vi "通道配置模块.vi"() -> (1 "返回":bool)   [LabVIEW 2010]
uses:
  全局量/试验配置信息.vi
  全局量/全局_配置.vi
  <vilib>/Utility/config.llb/Write Key (String).vi
  <vilib>/Utility/config.llb/NI_LVConfig.lvlib
panel:
  in  "str_IP":string
  in  "单选_LAN":bool
  in  "CAN波特率":T1(ring)
  in  "LAN端口":u32
  in  "RS485_2端口":refnum<visa-resource-name>="COM1"
  in  "RS485_1端口":refnum<visa-resource-name>="COM1"
  in  "RS485波特率":T2(ring)
  in  "R232端口":refnum<visa-resource-name>="COM1"
  out "配置文件路径":path
  out "配置文件目录":path
  in  "btn_保存配置":bool
  in  "加载配置文件列表":u16(ring)
  in  "保存配置文件名称":string
  in  "btn_返回":bool
  in  "选项卡控件":T3(tab)
  in  "CAN路数":u32=1 min=1 max=4
  in  "RS485路数":u32=1 min=1 max=1
  in  "RS232路数":u32=1 min=1 max=2
  in  "AD输入幅值":enum32{"±3V", "±5V", "±12V"}(ring)
  in  "AD输入路数":u32 min=1 max=16
  in  "DSP输入幅值":enum32{"0-3V"}(ring)
  in  "DSP输入路数":u32 min=1 max=16
  in  "数字量输入路数":u32 min=1 max=80
  in  "模拟量误差":dbl format="%.4f"
  in  "数字量输出路数":u32=1 min=1 max=76
  in  "D_IN_1":string[][](table) caption="表格"
  in  "D_IN_2":string[][](table) caption="表格"
  in  "D_IN_3":string[][](table) caption="表格"
  in  "D_IN_4":string[][](table) caption="表格"
  # "板卡测试配置"
  # "保存配置文件名称："
  # "加载配置文件："
  # "控制板IP："
  # "控制板端口："
  # "1号"
  # "COM端口："
  # "2号"
  # "COM端口："
  # "CAN总线通信波特率："
  # "RS485总线通信波特率："
  # "数字量输出信号路数："
  # "数字量输入信号路数："
  # "外部AD模拟量输入信号路数："
  # "DSP模拟量输入信号路数："
  # "外部AD模拟量输入信号幅值："
  # "DSP模拟量输入信号幅值："
  # "RS232总线通信路数："
  # "RS485总线通信路数："
  # "CAN总线通信路数："
  # "模拟量允许误差："
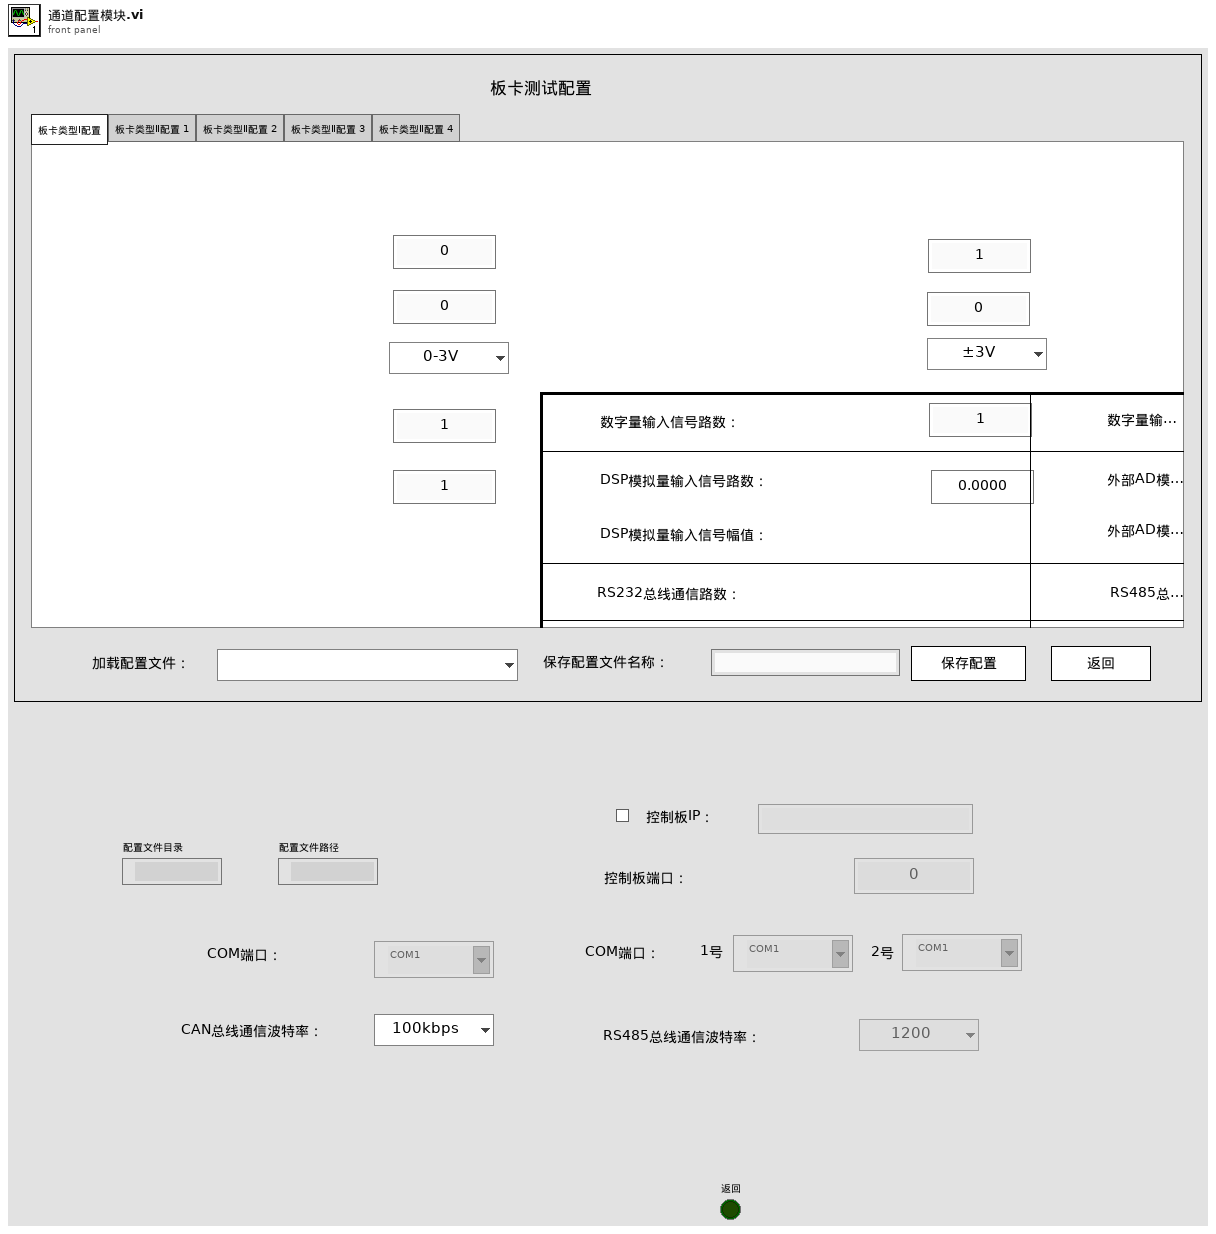
[diagram p1: front panel]
types:
  T1 = enum32{"100kbps", "200kbps", "250kbps", "500kbps", "1000kbps"}
  T2 = enum32{"1200", "2400", "4800", "9600", "19200", "57600", "115200", ""}
  T3 = enum32{"板卡类型Ⅰ配置", "板卡类型Ⅱ配置 1", "板卡类型Ⅱ配置 2", "板卡类型Ⅱ配置 3", "板卡类型Ⅱ配置 4"}
  T4 = enum8{"Enabled", "Disabled", "Disabled and Grayed Out"}
  T5 = cluster{"数字量输入路数":u32, "数字量输出路数":u32, "DSP输入路数":u32, "DSP输入幅值":enum32{"0-3V"}, "AD输入路数":u32, "AD输入幅值":enum32{"±3V", "±5V", "±12V"}, "毫秒倍数":u32, "RS232路数":u32, "模拟量误差":dbl, "毫秒倍数":u32, "RS485路数":u32, "RS485波特率":enum32{"1200", "2400", "4800", "9600", "19200", "57600", "115200", ""}, "CAN路数":u32, "CAN波特率":enum32{"100kbps", "200kbps", "250kbps", "500kbps", "1000kbps"}, "单选_LAN":bool, "str_IP":string, "LAN端口":u32}
  T6 = typedef "NI_LVConfig.lvlib/Config Data RefNum.ctl" = refnum<k1>
  T7 = cluster{"数字量输入信号路数":i32, "数字量输出信号路数":i32, "DSP模拟量输入信号路数":u32, "DSP模拟量输入信号幅值":u32, "AD模拟量输入信号路数":u32, "AD模拟量输入信号幅值":u32, "RS232端口":u32, "RS232通信路数":u32, "RS232波特率":dbl, "RS485端口":u32, "RS485通信路数":u32, "RS485波特率":u32, "CAN通信路数":i32, "CAN波特率":u32, "以太网选择?":bool, "控制板IP":string, "以太网端口":u32}
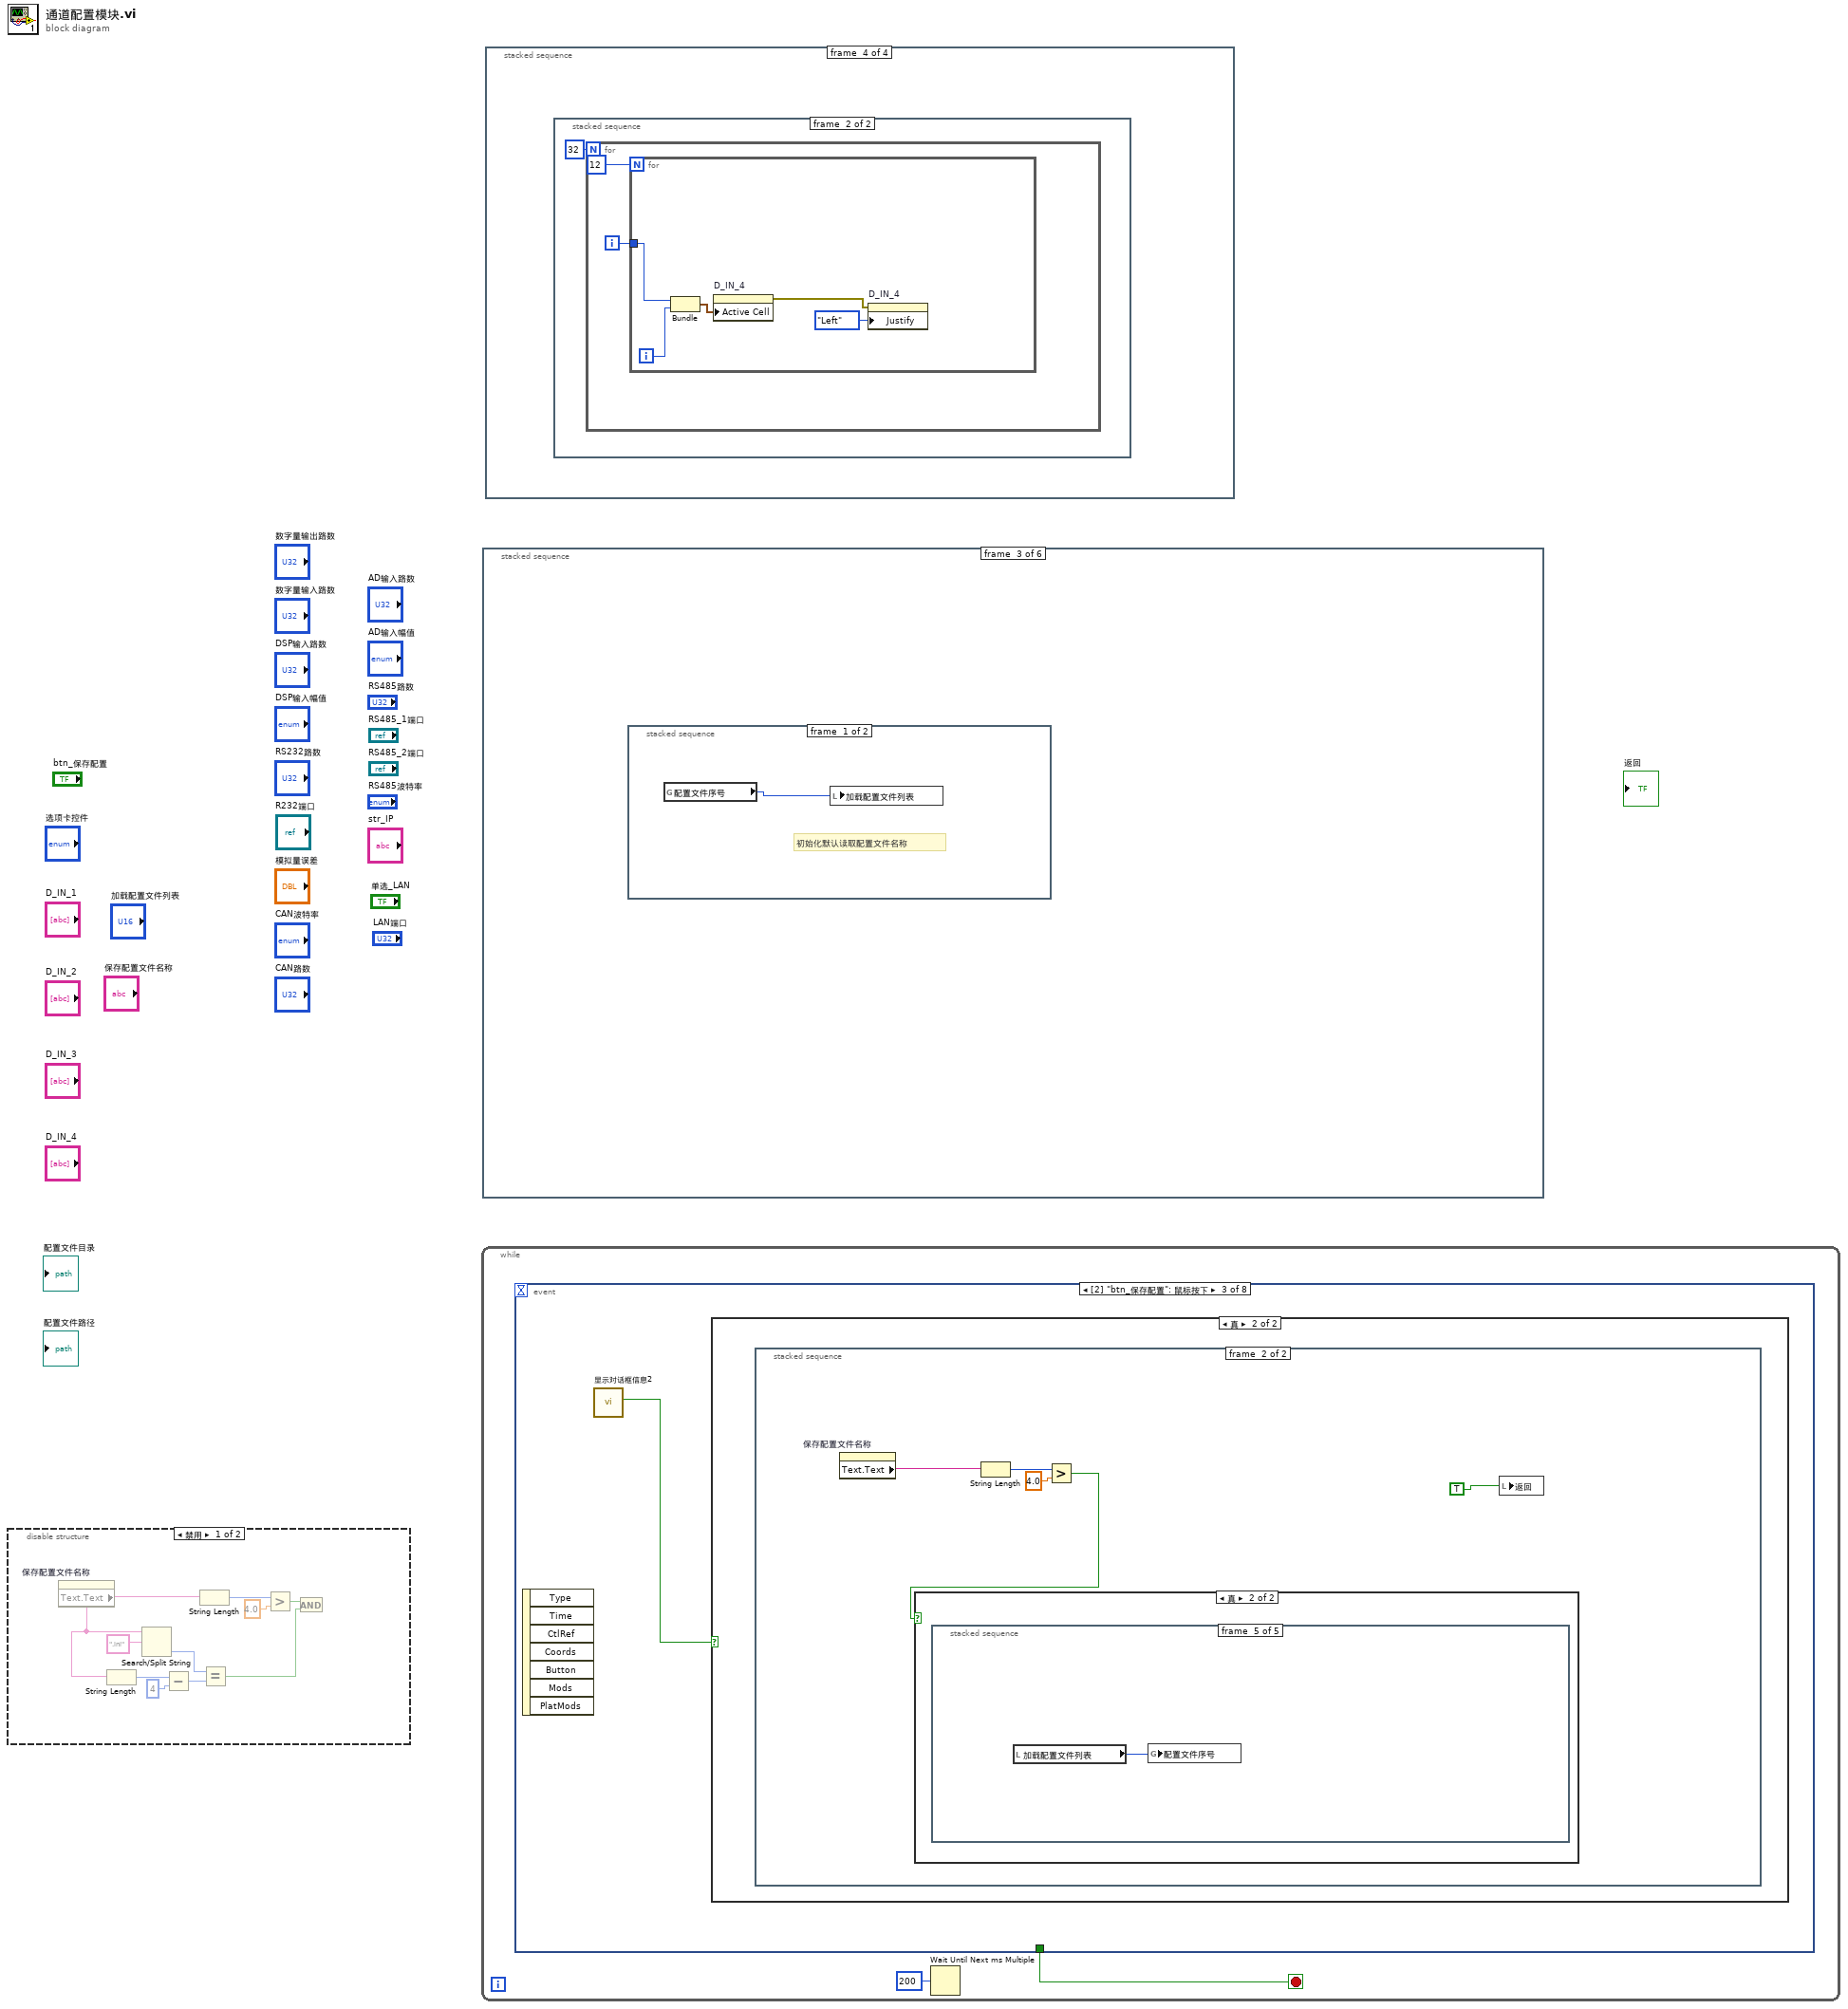
[diagram p0: block diagram]
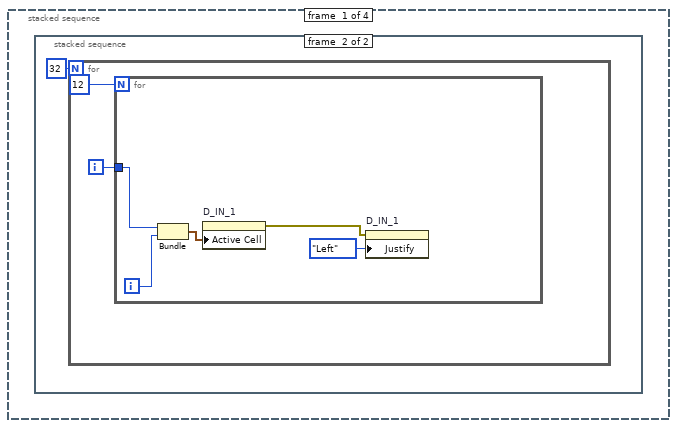
[diagram p2: hidden frame]
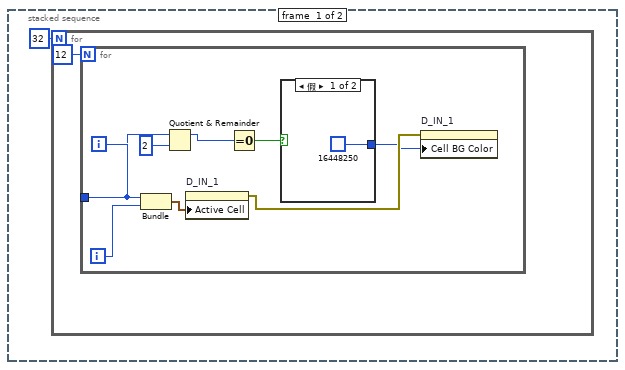
[diagram p3: hidden frame]
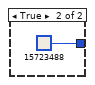
[diagram p4: hidden frame]
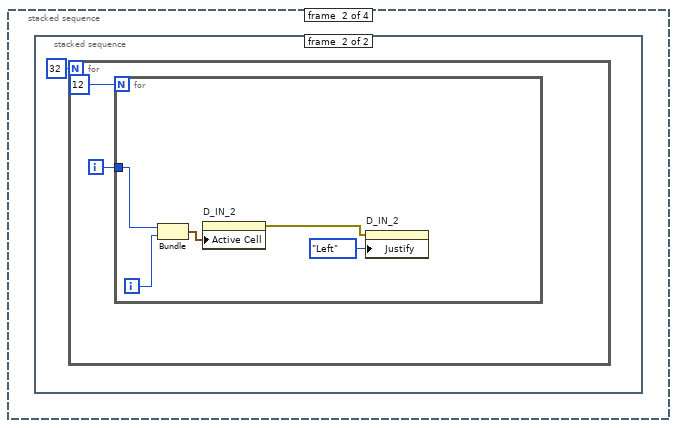
[diagram p5: hidden frame]
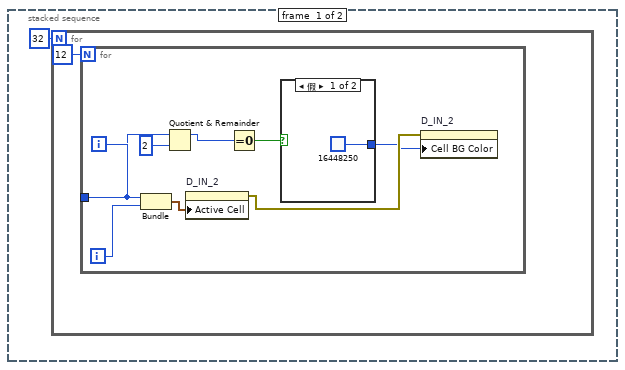
[diagram p6: hidden frame]
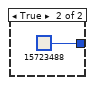
[diagram p7: hidden frame]
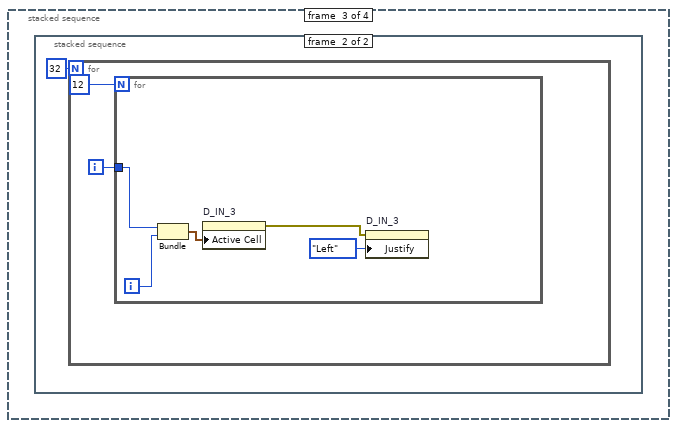
[diagram p8: hidden frame]
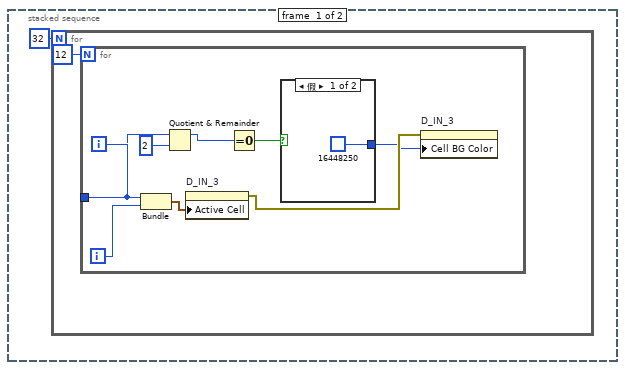
[diagram p9: hidden frame]
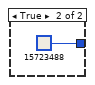
[diagram p10: hidden frame]
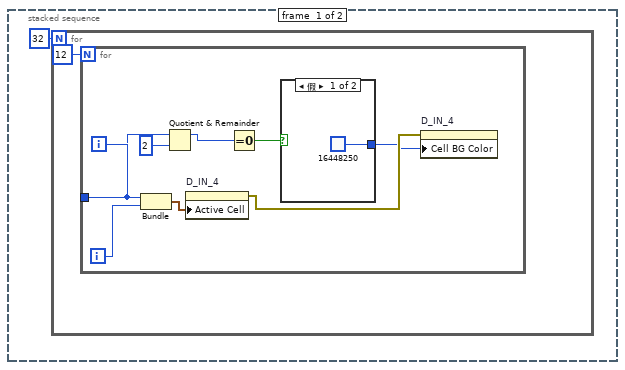
[diagram p11: hidden frame]
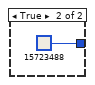
[diagram p12: hidden frame]
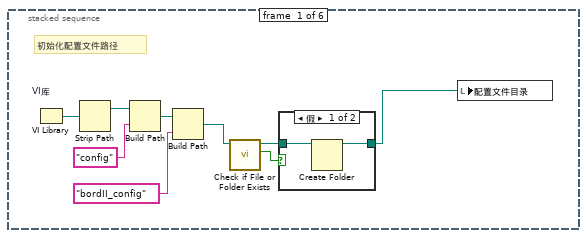
[diagram p14: hidden frame]
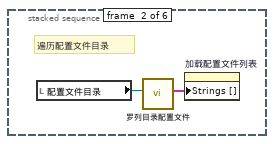
[diagram p16: hidden frame]
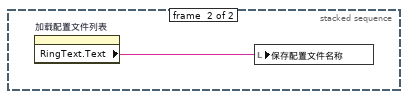
[diagram p17: hidden frame]
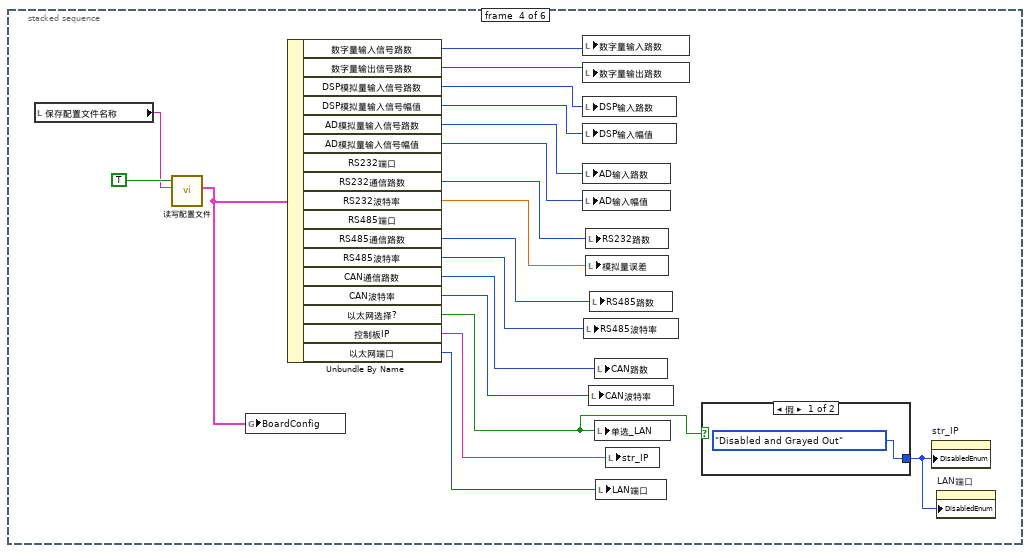
[diagram p18: hidden frame]
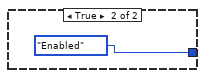
[diagram p19: hidden frame]
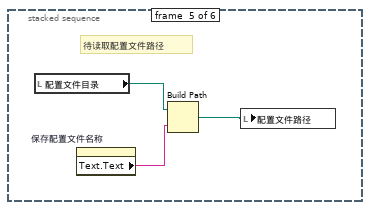
[diagram p20: hidden frame]
diagram:
  n1 = disable-structure shown="禁用" {
    frame Disabled {
      n2 = property on="保存配置文件名称" class="Str"() -> ("Text.Text"=w6:string)  [unwired: 2 in, 2 out]
      n3 = String Length(string=w6) -> (length=w7:i32)
      n4 = Search/Split String(string=w6, search string/char (-)=".ini" ("搜索字符串/字符(-)")) -> (offset of match=w5:i32)  [unwired: 1 in, 2 out]
      n5 = Subtract(x=w7, y=4) -> (x-y=w9:i32)
      n6 = String Length(string=w6) -> (length=w3:i32)
      n7 = Equal?(x=w5, y=w9) -> (x = y?=w10:bool)
      n8 = Greater?(x=w3, y=4.0) -> (0:w4:bool)
      n9 = And(x=w4, y=w10) -> ()  [unwired: 1 out]
    }
    frame Enabled {
    }
  }
  n10 = while {
    stop <- w12 stop-if-true
    n11 = event shown="[2] \"btn_保存配置\": 鼠标按下" {
      selector: _ -> [_ _ _ _ _ _ _ _]
      dyn-events: _ -> [_ _ _ _ _ _ _ _]
      timeout: _ -> [_ _ _ _ _ _ _ _]
      tunnel: [_ "btn_返回" _ _ _ _ _ TRUE] -> w12
      event Timeout {
        n12 = event-data() -> ()  [unwired: 1 in, 2 out]
      }
      event "btn_返回": Value Change {
        n13 = event-data() -> ()  [unwired: 1 in, 5 out]
      }
      event "btn_保存配置": Mouse Down {
        n14 = event-data() -> ()  [unwired: 1 in, 7 out]
        n15 = call "显示对话框信息2"() -> ("确定"=w14:bool)  [unwired: 10 in, 1 out]
        n16 = case shown="真" w14 {
          frame False {
          }
          frame True {
            n17 = stacked-sequence {
              frame #0 {
                n18 = local read "数字量输入路数"() -> (w22:u32)
                n19 = local read "数字量输出路数"() -> (w21:u32)
                n20 = local read "RS485波特率"() -> (w34:T2)
                n21 = local read "DSP输入路数"() -> (w20:u32)
                n22 = local read "DSP输入幅值"() -> (w25:enum32{"0-3V"})
                n23 = local read "模拟量误差"() -> (w23:dbl)
                n24 = local read "AD输入路数"() -> (w19:u32)
                n25 = local read "AD输入幅值"() -> (w24:enum32{"±3V", "±5V", "±12V"})
                n26 = local read "CAN波特率"() -> (w33:T1)
                n27 = local read "RS232路数"() -> (w18:u32)
                n28 = local read "RS485路数"() -> (w17:u32)
                n29 = local read "单选_LAN"() -> (w32:bool)
                n30 = local read "CAN路数"() -> (w16:u32)
                n31 = local read "LAN端口"() -> (w30:u32)
                n32 = local read "str_IP"() -> (w31:string)
                n33 = Bundle("数字量输入路数"=w22, "数字量输出路数"=w21, "DSP输入路数"=w20, "DSP输入幅值"=w25, "AD输入路数"=w19, "AD输入幅值"=w24, "毫秒倍数"=u32 0, "RS232路数"=w18, "模拟量误差"=w23, "毫秒倍数"=u32 0, "RS485路数"=w17, "RS485波特率"=w34, "CAN路数"=w16, "CAN波特率"=w33, "单选_LAN"=w32, "str_IP"=w31, "LAN端口"=w30) -> (w28:T5)  [unwired: 1 in]
                n34 = global write "全局_配置.vi" "BoardConfig"(w28) -> ()
                n35 = local read "保存配置文件名称"() -> (w15:string)
                n36 = call "读写配置文件.vi"("BoardConfig_input"=w28, "文件名称"=w15, "m_bRead"=FALSE) -> ()  [unwired: 8 in, 1 out]
                n37 = case shown="\"0-3V\", 默认" w25 {
                  tunnel: [3.3] -> w26
                  frame "0-3V", Default {
                  }
                }
                n38 = case shown="\"±12V\"" w24 {
                  tunnel: [6.0 10.0 24.0] -> w27
                  frame "±3V", Default {
                  }
                  frame "±5V" {
                  }
                  frame "±12V" {
                  }
                }
                n39 = global write "全局_配置.vi" "ad模拟量输入路数"(w19) -> ()
                n40 = global write "全局_配置.vi" "R232路数"(w18) -> ()
                n41 = global write "全局_配置.vi" "模拟量误差"(w23) -> ()
                n42 = global write "全局_配置.vi" "R485路数"(w17) -> ()
                n43 = global write "试验配置信息.vi" "自测CAN路数"(w16) -> ()
                n44 = global write "全局_配置.vi" "数字量输入路数"(w22) -> ()
                n45 = global write "全局_配置.vi" "数字量输出路数"(w21) -> ()
                n46 = global write "全局_配置.vi" "dsp模拟量输入路数"(w20) -> ()
                n47 = global write "全局_配置.vi" "DSP模拟量量程范围"(w26) -> ()
                n48 = global write "全局_配置.vi" "ARM模拟量量程范围"(w27) -> ()
              }
              frame #1 {
                n49 = property on="保存配置文件名称" class="Str"() -> ("Text.Text"=w43:string)  [unwired: 2 in, 2 out]
                n50 = String Length(string=w43) -> (length=w44:i32)
                n51 = Greater?(x=w44, y=4.0) -> (0:w42:bool)
                n52 = case shown="真" w42 {
                  frame False {
                    n53 = call "显示对话框信息"() -> ()  [unwired: 10 in, 2 out]
                  }
                  frame True {
                    n54 = stacked-sequence {
                      frame #0 {
                        # "待保存配置文件路径"
                        n55 = local read "配置文件目录"() -> (w48:path)
                        n56 = property on="保存配置文件名称" class="Str"() -> ("Text.Text"=w47:string)  [unwired: 2 in, 2 out]
                        n57 = Build Path(base path=w48, name or relative path=w47) -> (appended path=w46:path)
                        n58 = local write "配置文件路径"(w46) -> ()
                      }
                      frame #1 {
                        w65 = "TEST_CONFIG" ("key")
                        # "保存配置"
                        n59 = local read "D_IN_1"() -> (w67:string[][])
                        n60 = local read "配置文件路径"() -> (w76:path)
                        n61 = local read "D_IN_2"() -> (w68:string[][])
                        n62 = Array To Spreadsheet String(array=w67, 3:"%s" ("格式字符串")) -> (spreadsheet string=w70:string)  [unwired: 1 in]
                        n63 = call <vilib>:"Open Config Data.vi"("configuration file path"=w76) -> ("error out"=w75:errorcluster, "refnum"=w74:T6)  [unwired: 8 in, 1 out]
                        n64 = local read "D_IN_3"() -> (w56:string[][])
                        n65 = Array To Spreadsheet String(array=w68, 3:"%s" ("格式字符串")) -> (spreadsheet string=w66:string)  [unwired: 1 in]
                        n66 = call-poly <vilib>:"Write Key.vi"("section"=w65, "error in (no error)"=w75, "value"=w70, "key"="test1", "refnum"=w74) -> ("error out"=w73:errorcluster, "refnum out"=w72:T6)  [unwired: 4 in, 1 out]
                        n67 = local read "D_IN_4"() -> (w55:string[][])
                        n68 = Array To Spreadsheet String(array=w56, 3:"%s" ("格式字符串")) -> (spreadsheet string=w54:string)  [unwired: 1 in]
                        n69 = call-poly <vilib>:"Write Key.vi"("section"=w65, "error in (no error)"=w73, "value"=w66, "key"="test2", "refnum"=w72) -> ("error out"=w61:errorcluster, "refnum out"=w64:T6)  [unwired: 4 in, 1 out]
                        n70 = Array To Spreadsheet String(array=w55, 3:"%s" ("格式字符串")) -> (spreadsheet string=w53:string)  [unwired: 1 in]
                        n71 = call-poly <vilib>:"Write Key.vi"("section"=w65, "error in (no error)"=w61, "value"=w54, "key"="test3", "refnum"=w64) -> ("error out"=w60:errorcluster, "refnum out"=w63:T6)  [unwired: 4 in, 1 out]
                        n72 = call-poly <vilib>:"Write Key.vi"("section"=w65, "error in (no error)"=w60, "value"=w53, "key"="test4", "refnum"=w63) -> ("error out"=w59:errorcluster, "refnum out"=w62:T6)  [unwired: 4 in, 1 out]
                        n73 = call <vilib>:"Close Config Data.vi"("error in (no error)"=w59, "refnum"=w62) -> ()  [unwired: 8 in, 2 out]
                      }
                      frame #2 {
                        # "刷新下拉列表"
                        n74 = local read "配置文件目录"() -> (w78:path)
                        n75 = call "罗列目录配置文件.vi"("路径"=w78) -> ("数组"=w77:string[])  [unwired: 10 in]
                        n76 = property on="加载配置文件列表" class="Ring (严格)"("Strings []"=w77) -> ()  [unwired: 2 in, 2 out]
                      }
                      frame #3 {
                        # "选中当前配置文件"
                        n77 = property on="保存配置文件名称" class="Str"() -> ("Text.Text"=w79:string)  [unwired: 2 in, 2 out]
                        n78 = property on="加载配置文件列表" class="Ring (严格)"("RingText.Text"=w79) -> ()  [unwired: 2 in, 2 out]
                      }
                      frame #4 {
                        n79 = local read "加载配置文件列表"() -> (w80:u16)
                        n80 = global write "试验配置信息.vi" "配置文件序号"(w80) -> ()
                      }
                    }
                  }
                }
                n81 = local write "返回"(TRUE) -> ()
              }
            }
          }
        }
      }
      event "单选_LAN": Value Change {
        n82 = event-data() -> ("NewVal"=w81:bool)  [unwired: 1 in, 4 out]
        n83 = case shown="假" w81 {
          tunnel: [T4."Disabled and Grayed Out" ("禁用") T4."Enabled" ("禁用")] -> w82
          frame False {
          }
          frame True {
          }
        }
        n84 = property on="str_IP" class="Str"("DisabledEnum"=w82) -> ()  [unwired: 2 in, 2 out]
        n85 = property on="LAN端口" class="DigNum (严格)"("DisabledEnum"=w82) -> ()  [unwired: 2 in, 2 out]
      }
      event "RS485路数": Value Change {
        n86 = event-data() -> ()  [unwired: 1 in, 5 out]
        n87 = disable-structure shown="禁用" {
          frame Disabled {
            n88 = case shown="\"1\"" {
              selector: _ -> [_ _]
              tunnel: [w87 T4."Disabled" ("禁用")] -> w86
              tunnel: [w87 T4."Disabled" ("禁用")] -> w85
              tunnel: [w87 T4."Disabled and Grayed Out" ("禁用")] -> _
              frame "1", Default {
                w87 = T4."Disabled and Grayed Out" ("禁用")
              }
              frame "1" {
              }
            }
            n89 = property on="RS485波特率" class="Enum (严格)"("DisabledEnum"=w85) -> ()  [unwired: 2 in, 2 out]
            n90 = property on="RS485_1端口" class="VISAName"("DisabledEnum"=w86) -> ()  [unwired: 2 in, 2 out]
          }
          frame Enabled {
          }
        }
      }
      event "RS232路数": Value Change {
        n91 = event-data() -> ()  [unwired: 1 in, 5 out]
        n92 = disable-structure shown="禁用" {
          frame Disabled {
            n93 = case shown="\"1\"" {
              selector: _ -> [_ _]
              tunnel: [T4."Disabled and Grayed Out" ("禁用") T4."Enabled" ("禁用")] -> w91
              frame "1", Default {
              }
              frame "1" {
              }
            }
            n94 = property on="R232端口" class="VISAName"("DisabledEnum"=w91) -> ()  [unwired: 2 in, 2 out]
          }
          frame Enabled {
          }
        }
      }
      event "加载配置文件列表": Value Change {
        n95 = event-data() -> ()  [unwired: 1 in, 5 out]
        n96 = stacked-sequence {
          frame #0 {
            n97 = property on="加载配置文件列表" class="Ring (严格)"() -> ("RingText.Text"=w94:string)  [unwired: 2 in, 2 out]
            n98 = local write "保存配置文件名称"(w94) -> ()
          }
          frame #1 {
            n99 = local read "保存配置文件名称"() -> (w112:string)
            n100 = call "读写配置文件.vi"("文件名称"=w112, "m_bRead"=TRUE) -> ("BoardConfig_output"=w95:T7)  [unwired: 9 in]
            n101 = global write "全局_配置.vi" "BoardConfig"(w95) -> ()
            n102 = Unbundle By Name(w95) -> ("数字量输入信号路数"=w96:i32, "数字量输出信号路数"=w97:i32, "DSP模拟量输入信号路数"=w101:u32, "DSP模拟量输入信号幅值"=w98:u32, "AD模拟量输入信号路数"=w99:u32, "AD模拟量输入信号幅值"=w100:u32, "RS232通信路数"=w102:u32, "RS232波特率"=w103:dbl, "RS485通信路数"=w104:u32, "RS485波特率"=w105:u32, "CAN通信路数"=w106:i32, "CAN波特率"=w107:u32, "以太网选择?"=w110:bool, "控制板IP"=w108:string, "以太网端口"=w109:u32)  [unwired: 2 out]
            n103 = local write "数字量输入路数"(w96) -> ()
            n104 = local write "数字量输出路数"(w97) -> ()
            n105 = local write "DSP输入路数"(w101) -> ()
            n106 = local write "DSP输入幅值"(w98) -> ()
            n107 = local write "AD输入路数"(w99) -> ()
            n108 = local write "AD输入幅值"(w100) -> ()
            n109 = local write "RS485波特率"(w105) -> ()
            n110 = local write "RS232路数"(w102) -> ()
            n111 = local write "模拟量误差"(w103) -> ()
            n112 = local write "CAN波特率"(w107) -> ()
            n113 = local write "RS485路数"(w104) -> ()
            n114 = local write "CAN路数"(w106) -> ()
            n115 = local write "单选_LAN"(w110) -> ()
            n116 = local write "LAN端口"(w109) -> ()
            n117 = local write "str_IP"(w108) -> ()
            n118 = case shown="假" w110 {
              tunnel: [T4."Disabled and Grayed Out" ("禁用") T4."Enabled" ("禁用")] -> w111
              frame False {
              }
              frame True {
              }
            }
            n119 = property on="str_IP" class="Str"("DisabledEnum"=w111) -> ()  [unwired: 2 in, 2 out]
            n120 = property on="LAN端口" class="DigNum (严格)"("DisabledEnum"=w111) -> ()  [unwired: 2 in, 2 out]
          }
          frame #2 {
            n121 = local read "配置文件目录"() -> (w118:path)
            n122 = property on="保存配置文件名称" class="Str"() -> ("Text.Text"=w117:string)  [unwired: 2 in, 2 out]
            n123 = Build Path(base path=w118, name or relative path=w117) -> (appended path=w116:path)
            n124 = local write "配置文件路径"(w116) -> ()
          }
          frame #3 {
            n125 = local read "配置文件路径"() -> (w119:path)
            n126 = call "函数测试配置文件读取.vi"("配置文件路径"=w119) -> ("D_IN_4"=w123:string[][], "D_IN_3"=w122:string[][], "D_IN_2"=w121:string[][], "D_IN_1"=w120:string[][])  [unwired: 6 in]
            n127 = local write "D_IN_2"(w121) -> ()
            n128 = local write "D_IN_3"(w122) -> ()
            n129 = local write "D_IN_4"(w123) -> ()
            n130 = local write "D_IN_1"(w120) -> ()
          }
        }
      }
      event Panel Close {
        n131 = event-data() -> ()  [unwired: 1 in, 3 out]
      }
    }
    n132 = Wait Until Next ms Multiple(millisecond multiple=u32 200 ("毫秒倍数")) -> ()  [unwired: 1 out]
  }
  n133 = stacked-sequence {
    frame #0 {
      # "初始化配置文件路径"
      n134 = VI Library "VI库"() -> (path=w133:path)
      n135 = Strip Path(path=w133) -> (stripped path=w132:path)  [unwired: 1 out]
      n136 = Build Path(base path=w132, name or relative path="config" ("名称或相对路径")) -> (appended path=w130:path)
      n137 = Build Path(base path=w130, name or relative path="bordII_config" ("名称或相对路径")) -> (appended path=w126:path)
      n138 = call <vilib>:"Check if File or Folder Exists.vi"("path"=w126) -> ("file or folder exists?"=w127:bool, "dup path"=w128:path)  [unwired: 8 in, 1 out]
      n139 = case shown="假" w127 {
        tunnel: w128 -> [w134 w136]
        tunnel: [w135 w136] -> w125
        frame False {
          n140 = Create Folder(path (use dialog)=w134) -> (created path=w135:path)  [unwired: 2 in, 2 out]
        }
        frame True {
        }
      }
      n141 = local write "配置文件目录"(w125) -> ()
    }
    frame #1 {
      # "遍历配置文件目录"
      n142 = local read "配置文件目录"() -> (w137:path)
      n143 = call "罗列目录配置文件.vi"("路径"=w137) -> ("数组"=w138:string[])  [unwired: 10 in]
      n144 = property on="加载配置文件列表" class="Ring (严格)"("Strings []"=w138) -> ()  [unwired: 2 in, 2 out]
    }
    frame #2 {
      n145 = stacked-sequence {
        frame #0 {
          # "初始化默认读取配置文件名称"
          n146 = global read "试验配置信息.vi" "配置文件序号"() -> (w139:u16)
          n147 = local write "加载配置文件列表"(w139) -> ()
        }
        frame #1 {
          n148 = property on="加载配置文件列表" class="Ring (严格)"() -> ("RingText.Text"=w140:string)  [unwired: 2 in, 2 out]
          n149 = local write "保存配置文件名称"(w140) -> ()
        }
      }
    }
    frame #3 {
      n150 = local read "保存配置文件名称"() -> (w158:string)
      n151 = call "读写配置文件.vi"("文件名称"=w158, "m_bRead"=TRUE) -> ("BoardConfig_output"=w141:T7)  [unwired: 9 in]
      n152 = global write "全局_配置.vi" "BoardConfig"(w141) -> ()
      n153 = Unbundle By Name(w141) -> ("数字量输入信号路数"=w157:i32, "数字量输出信号路数"=w156:i32, "DSP模拟量输入信号路数"=w152:u32, "DSP模拟量输入信号幅值"=w155:u32, "AD模拟量输入信号路数"=w154:u32, "AD模拟量输入信号幅值"=w153:u32, "RS232通信路数"=w151:u32, "RS232波特率"=w150:dbl, "RS485通信路数"=w149:u32, "RS485波特率"=w148:u32, "CAN通信路数"=w147:i32, "CAN波特率"=w146:u32, "以太网选择?"=w143:bool, "控制板IP"=w145:string, "以太网端口"=w144:u32)  [unwired: 2 out]
      n154 = local write "数字量输入路数"(w157) -> ()
      n155 = local write "数字量输出路数"(w156) -> ()
      n156 = local write "DSP输入路数"(w152) -> ()
      n157 = local write "DSP输入幅值"(w155) -> ()
      n158 = local write "AD输入路数"(w154) -> ()
      n159 = local write "AD输入幅值"(w153) -> ()
      n160 = local write "RS485波特率"(w148) -> ()
      n161 = local write "RS232路数"(w151) -> ()
      n162 = local write "模拟量误差"(w150) -> ()
      n163 = local write "CAN波特率"(w146) -> ()
      n164 = local write "RS485路数"(w149) -> ()
      n165 = local write "CAN路数"(w147) -> ()
      n166 = local write "单选_LAN"(w143) -> ()
      n167 = local write "LAN端口"(w144) -> ()
      n168 = local write "str_IP"(w145) -> ()
      n169 = case shown="假" w143 {
        tunnel: [T4."Disabled and Grayed Out" ("禁用") T4."Enabled" ("禁用")] -> w142
        frame False {
        }
        frame True {
        }
      }
      n170 = property on="str_IP" class="Str"("DisabledEnum"=w142) -> ()  [unwired: 2 in, 2 out]
      n171 = property on="LAN端口" class="DigNum (严格)"("DisabledEnum"=w142) -> ()  [unwired: 2 in, 2 out]
    }
    frame #4 {
      # "待读取配置文件路径"
      n172 = local read "配置文件目录"() -> (w163:path)
      n173 = property on="保存配置文件名称" class="Str"() -> ("Text.Text"=w162:string)  [unwired: 2 in, 2 out]
      n174 = Build Path(base path=w163, name or relative path=w162) -> (appended path=w164:path)
      n175 = local write "配置文件路径"(w164) -> ()
    }
    frame #5 {
      # "读取默认配置的配置内容"
      n176 = local read "配置文件路径"() -> (w169:path)
      n177 = call "函数测试配置文件读取.vi"("配置文件路径"=w169) -> ("D_IN_4"=w165:string[][], "D_IN_3"=w166:string[][], "D_IN_2"=w167:string[][], "D_IN_1"=w168:string[][])  [unwired: 6 in]
      n178 = local write "D_IN_2"(w167) -> ()
      n179 = local write "D_IN_3"(w166) -> ()
      n180 = local write "D_IN_4"(w165) -> ()
      n181 = local write "D_IN_1"(w168) -> ()
    }
  }
  n182 = stacked-sequence {
    frame #0 {
      n183 = stacked-sequence {
        frame #0 {
          n184 = for {
            N: 32 -> [_]
            i -> [w172]
            n185 = for {
              N: 12 -> [_]
              tunnel: w172 -> [w179]
              i -> [w173]
              n186 = Bundle(w179, w173) -> (w176:cluster{i32, i32})  [unwired: 1 in]
              n187 = Quotient & Remainder(x=w179, y=2) -> (x-y*floor(x/y)=w177:i32)  [unwired: 1 out]
              n188 = property on="D_IN_1" class="Tbl (严格)"("Active Cell"=w176) -> (error out=w175:errorcluster)  [unwired: 2 in, 1 out]
              n189 = Equal To 0?(x=w177) -> (x = 0?=w180:bool)
              n190 = case shown="假" w180 {
                tunnel: [u32 16448250 u32 15723488] -> w174
                frame False {
                }
                frame True {
                }
              }
              n191 = property on="D_IN_1" class="Tbl (严格)"(error in=w175, "Cell BG Color"=w174) -> ()  [unwired: 1 in, 2 out]
            }
          }
        }
        frame #1 {
          n192 = for {
            N: 32 -> [_]
            i -> [w184]
            n193 = for {
              N: 12 -> [_]
              tunnel: w184 -> [w186]
              i -> [w187]
              n194 = Bundle(w186, w187) -> (w190:cluster{i32, i32})  [unwired: 1 in]
              n195 = property on="D_IN_1" class="Tbl (严格)"("Active Cell"=w190) -> (error out=w188:errorcluster)  [unwired: 2 in, 1 out]
              n196 = property on="D_IN_1" class="Tbl (严格)"(error in=w188, "Justify"=enum16{"Left", "Center", "Right"}."Left" ("活动单元格:单元格对齐")) -> ()  [unwired: 1 in, 2 out]
            }
          }
        }
      }
    }
    frame #1 {
      n197 = stacked-sequence {
        frame #0 {
          n198 = for {
            N: 32 -> [_]
            i -> [w193]
            n199 = for {
              N: 12 -> [_]
              tunnel: w193 -> [w200]
              i -> [w194]
              n200 = Bundle(w200, w194) -> (w197:cluster{i32, i32})  [unwired: 1 in]
              n201 = Quotient & Remainder(x=w200, y=2) -> (x-y*floor(x/y)=w198:i32)  [unwired: 1 out]
              n202 = property on="D_IN_2" class="Tbl (严格)"("Active Cell"=w197) -> (error out=w196:errorcluster)  [unwired: 2 in, 1 out]
              n203 = Equal To 0?(x=w198) -> (x = 0?=w201:bool)
              n204 = case shown="假" w201 {
                tunnel: [u32 16448250 u32 15723488] -> w195
                frame False {
                }
                frame True {
                }
              }
              n205 = property on="D_IN_2" class="Tbl (严格)"(error in=w196, "Cell BG Color"=w195) -> ()  [unwired: 1 in, 2 out]
            }
          }
        }
        frame #1 {
          n206 = for {
            N: 32 -> [_]
            i -> [w205]
            n207 = for {
              N: 12 -> [_]
              tunnel: w205 -> [w207]
              i -> [w208]
              n208 = Bundle(w207, w208) -> (w211:cluster{i32, i32})  [unwired: 1 in]
              n209 = property on="D_IN_2" class="Tbl (严格)"("Active Cell"=w211) -> (error out=w209:errorcluster)  [unwired: 2 in, 1 out]
              n210 = property on="D_IN_2" class="Tbl (严格)"(error in=w209, "Justify"=enum16{"Left", "Center", "Right"}."Left" ("活动单元格:单元格对齐")) -> ()  [unwired: 1 in, 2 out]
            }
          }
        }
      }
    }
    frame #2 {
      n211 = stacked-sequence {
        frame #0 {
          n212 = for {
            N: 32 -> [_]
            i -> [w214]
            n213 = for {
              N: 12 -> [_]
              tunnel: w214 -> [w221]
              i -> [w215]
              n214 = Bundle(w221, w215) -> (w218:cluster{i32, i32})  [unwired: 1 in]
              n215 = Quotient & Remainder(x=w221, y=2) -> (x-y*floor(x/y)=w219:i32)  [unwired: 1 out]
              n216 = property on="D_IN_3" class="Tbl (严格)"("Active Cell"=w218) -> (error out=w217:errorcluster)  [unwired: 2 in, 1 out]
              n217 = Equal To 0?(x=w219) -> (x = 0?=w222:bool)
              n218 = case shown="假" w222 {
                tunnel: [u32 16448250 u32 15723488] -> w216
                frame False {
                }
                frame True {
                }
              }
              n219 = property on="D_IN_3" class="Tbl (严格)"(error in=w217, "Cell BG Color"=w216) -> ()  [unwired: 1 in, 2 out]
            }
          }
        }
        frame #1 {
          n220 = for {
            N: 32 -> [_]
            i -> [w226]
            n221 = for {
              N: 12 -> [_]
              tunnel: w226 -> [w228]
              i -> [w229]
              n222 = Bundle(w228, w229) -> (w232:cluster{i32, i32})  [unwired: 1 in]
              n223 = property on="D_IN_3" class="Tbl (严格)"("Active Cell"=w232) -> (error out=w230:errorcluster)  [unwired: 2 in, 1 out]
              n224 = property on="D_IN_3" class="Tbl (严格)"(error in=w230, "Justify"=enum16{"Left", "Center", "Right"}."Left" ("活动单元格:单元格对齐")) -> ()  [unwired: 1 in, 2 out]
            }
          }
        }
      }
    }
    frame #3 {
      n225 = stacked-sequence {
        frame #0 {
          n226 = for {
            N: 32 -> [_]
            i -> [w235]
            n227 = for {
              N: 12 -> [_]
              tunnel: w235 -> [w242]
              i -> [w236]
              n228 = Bundle(w242, w236) -> (w239:cluster{i32, i32})  [unwired: 1 in]
              n229 = Quotient & Remainder(x=w242, y=2) -> (x-y*floor(x/y)=w240:i32)  [unwired: 1 out]
              n230 = property on="D_IN_4" class="Tbl (严格)"("Active Cell"=w239) -> (error out=w238:errorcluster)  [unwired: 2 in, 1 out]
              n231 = Equal To 0?(x=w240) -> (x = 0?=w243:bool)
              n232 = case shown="假" w243 {
                tunnel: [u32 16448250 u32 15723488] -> w237
                frame False {
                }
                frame True {
                }
              }
              n233 = property on="D_IN_4" class="Tbl (严格)"(error in=w238, "Cell BG Color"=w237) -> ()  [unwired: 1 in, 2 out]
            }
          }
        }
        frame #1 {
          n234 = for {
            N: 32 -> [_]
            i -> [w247]
            n235 = for {
              N: 12 -> [_]
              tunnel: w247 -> [w249]
              i -> [w250]
              n236 = Bundle(w249, w250) -> (w253:cluster{i32, i32})  [unwired: 1 in]
              n237 = property on="D_IN_4" class="Tbl (严格)"("Active Cell"=w253) -> (error out=w251:errorcluster)  [unwired: 2 in, 1 out]
              n238 = property on="D_IN_4" class="Tbl (严格)"(error in=w251, "Justify"=enum16{"Left", "Center", "Right"}."Left" ("活动单元格:单元格对齐")) -> ()  [unwired: 1 in, 2 out]
            }
          }
        }
      }
    }
  }
